vi "FP Position.vi"(11 "This VI":refnum<vi>) -> ()   [LabVIEW 2021, in "Master.lvlib"]
uses:
  Master.lvlib
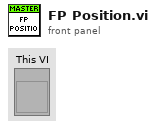
[diagram p1: front panel]
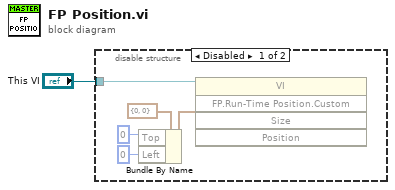
[diagram p0: block diagram]
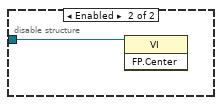
[diagram p2: hidden frame]
diagram:
  n1 = disable-structure shown="Disabled" {
    disable-tunnel: "This VI" -> [w6 w7]
    frame Disabled {
      n2 = Bundle By Name(cluster=cluster{"Top":i16, "Left":i16} {"Top"=0, "Left"=0} ("Position"), "Top"=i16 0, "Left"=i16 0) -> (w4:cluster{"Top":i16, "Left":i16})
      n3 = invoke class="VI" method="FP.Run-Time Position.Custom"(reference=w6, "Size"=w4) -> ()  [unwired: 3 in, 5 out]
    }
    frame Enabled {
      n4 = invoke class="VI" method="FP.Center"(reference=w7) -> ()  [unwired: 2 in, 3 out]
    }
  }
